vi "Start Sync.vi"(8 "error in (no error)":errorcluster, 10 "current time":timestamp, 11 "gRPC Server in":refnum<class "HVC3.lvclass">) -> (0 "error out":errorcluster, 3 "gRPC Server out":refnum<class "HVC3.lvclass">)   [LabVIEW 2019, in "HVC3.lvlib" / "HVC3.lvclass"]
uses:
  HVC3.lvclass
  RPC Messages/measurementservice_DMMConfigRequest/measurementservice_DMMConfigRequest_Data.ctl
  HVC3.lvclass/HVC3.ctl
  RPC Messages/measurementservice_QueryResponse/measurementservice_QueryResponse_Data.ctl
  RPC Messages/measurementservice_DMMConfigResponse/measurementservice_DMMConfigResponse_Data.ctl
  RPC Messages/measurementservice_ErrorOut/measurementservice_ErrorOut_Data.ctl
  RPC Messages/measurementservice_DMMVoltageData/measurementservice_DMMVoltageData_Data.ctl
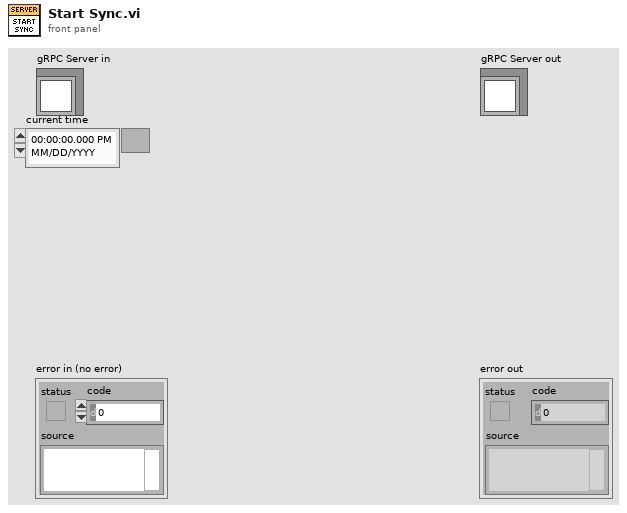
[diagram p1: front panel]
types:
  T1 = typedef "HVC3.lvlib/HVC3.lvclass/measurementservice_DMMConfigRequest_Data.ctl" = cluster{"DMMFunction":i32, "DMMResolution":sgl, "DMMRange":sgl, "DMMSampleCount":i32, "DMMApertureTimeUnit":i32, "DMMApertureTime":sgl, "DMMNumberofAverages":i32, "DMMAutoZero":i32, "DMMADCCalibration":i32, "DMMSettleTime":sgl}
  T2 = cluster{"measurementservice_DMMConfigRequest_Data":T1}
  T3 = typedef "HVC3.lvlib/HVC3.lvclass/measurementservice_QueryResponse_Data.ctl" = cluster{"message":string, "status":i32}
  T4 = typedef "HVC3.lvlib/HVC3.lvclass/measurementservice_ErrorOut_Data.ctl" = cluster{"errCode":i32, "errMessage":string}
  T5 = typedef "HVC3.lvlib/HVC3.lvclass/measurementservice_DMMConfigResponse_Data.ctl" = cluster{"DMMFunction":i32, "DMMResolution":sgl, "DMMRange":sgl, "DMMSampleCount":i32, "DMMApertureTimeUnit":i32, "DMMApertureTime":sgl, "DMMNumberofAverages":i32, "DMMAutoZero":i32, "DMMADCCalibration":i32, "DMMSettleTime":sgl, "error":T4}
  T6 = typedef "HVC3.lvlib/HVC3.lvclass/measurementservice_DMMVoltageData_Data.ctl" = cluster{"voltage":sgl[], "error":T4}
  T7 = typedef "HVC3.lvlib/HVC3.lvclass/Server gRPC UEs.ctl" = cluster{"Invoke gRPC UE":refnum<user-event>, "Query gRPC UE":refnum<user-event>, "Register gRPC UE":refnum<user-event>, "ConfigureDMM gRPC UE":refnum<user-event>, "PerformDMMVoltageMeasurement gRPC UE":refnum<user-event>}
  T8 = typedef "HVC3.lvlib/gprc-lvsupport.lvlib/grpcId.ctl" = u64
  T9 = typedef "HVC3.lvlib/HVC3.lvclass/measurementservice_QueryRequest_Data.ctl" = cluster{"query":string}
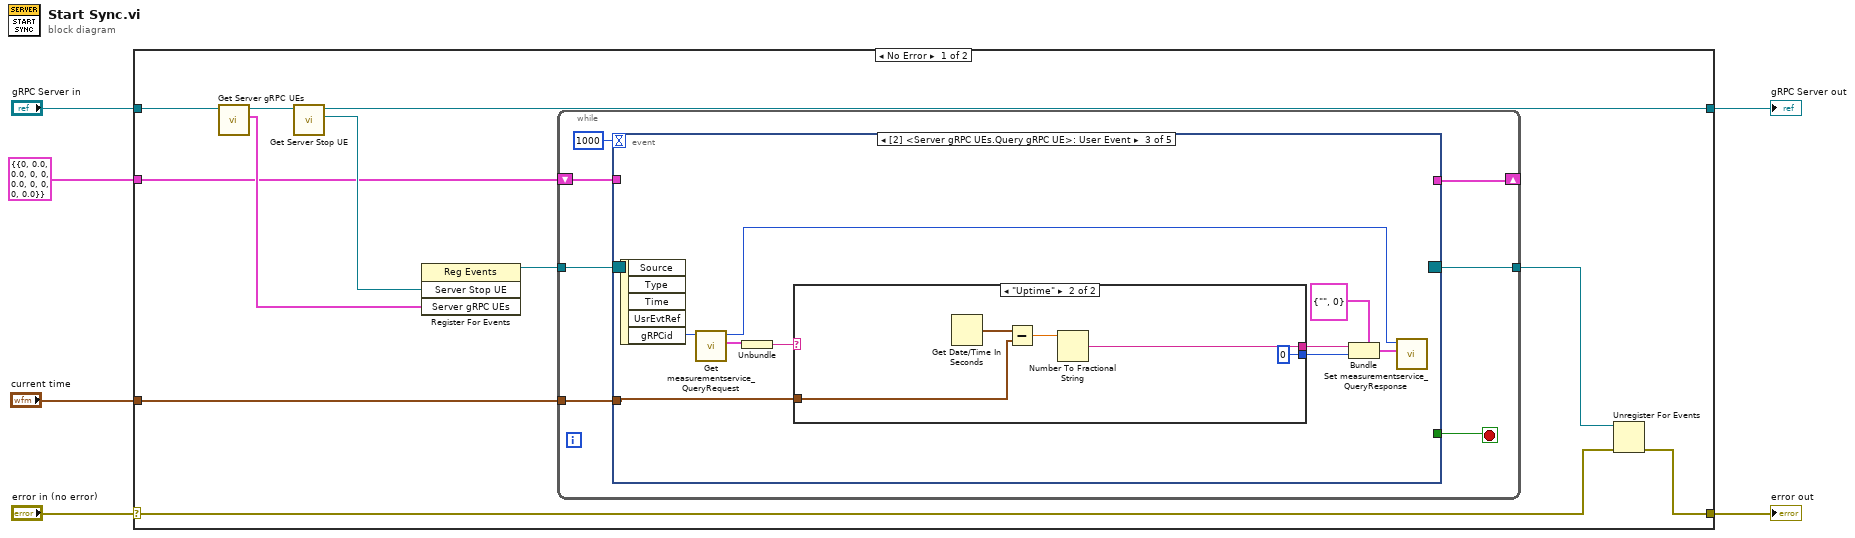
[diagram p0: block diagram]
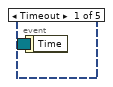
[diagram p2: hidden frame]
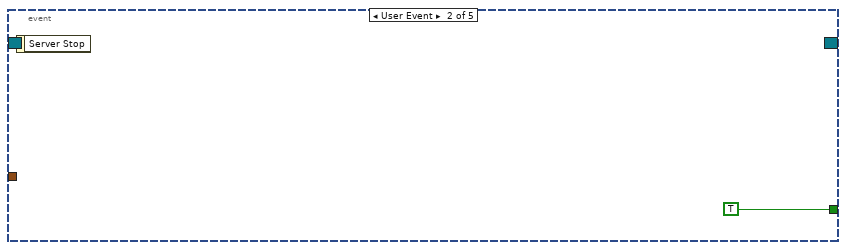
[diagram p3: hidden frame]
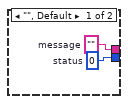
[diagram p4: hidden frame]
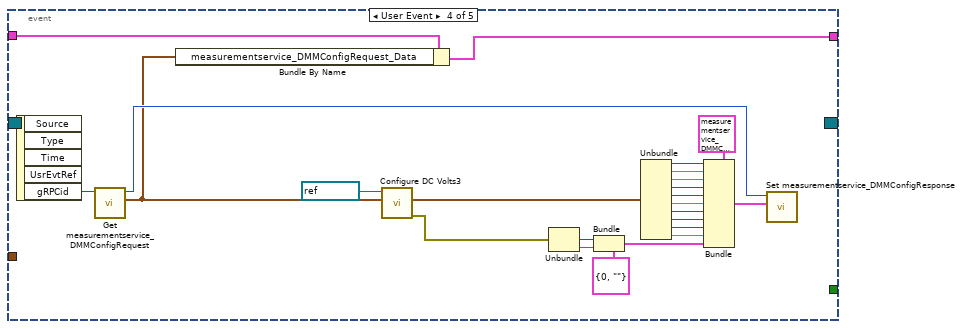
[diagram p5: hidden frame]
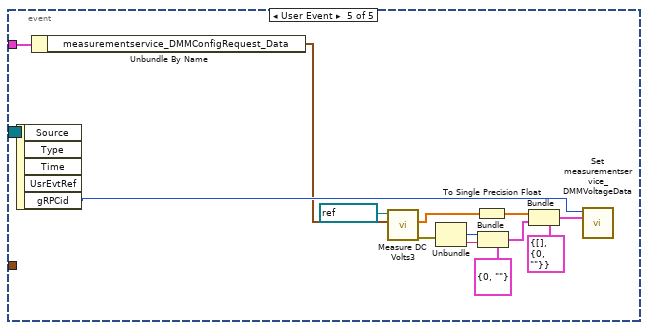
[diagram p6: hidden frame]
diagram:
  n1 = case shown="No Error" "error in (no error)" {
    selector: "error in (no error)" -> [w10 w80]
    tunnel: [w9 w80] -> w5
    tunnel: [w13 w79] -> w3
    tunnel: "gRPC Server in" -> [w17 w79]
    tunnel: "current time" -> [w8 _]
    tunnel: T2 {"measurementservice_DMMConfigRequest_Data"={"DMMFunction"=0, "DMMResolution"=0.0, "DMMRange"=0.0, "DMMSampleCount"=0, "DMMApertureTimeUnit"=0, "DMMApertureTime"=0.0, "DMMNumberofAverages"=0, "DMMAutoZero"=0, "DMMADCCalibration"=0, "DMMSettleTime"=0.0}} -> [w7 _]
    frame No Error {
      n2 = call "Get Server gRPC UEs.vi"("OOP Server in"=w17) -> ("Server gRPC UEs"=w14:T7, "OOP Server out"=w16:refnum<class "HVC3.lvclass">)  [unwired: 9 in]
      n3 = call "Get Server Stop UE.vi"("OOP Server in"=w16) -> ("Server Stop UE"=w15:refnum<user-event>, "OOP Server out"=w13:refnum<class "HVC3.lvclass">)  [unwired: 9 in]
      n4 = register-events(w15, w14) -> (reference out=w12:refnum<event-registration>)  [unwired: 2 in, 1 out]
      n5 = while {
        tunnel: w12 -> [w24]
        tunnel: [w22] -> w11
        tunnel: w8 -> [w20]
        shift-right: [w18] -> _
        shift-left: w7 -> [w19]
        stop <- w23 stop-if-true
        n6 = event "RPC Methods Event Structure" shown="[2] <Server gRPC UEs.Query gRPC UE>: User Event" {
          selector: w24 -> [_ _ _ _ _]
          dyn-events: [_ _ _ _ _] -> w22
          timeout: 1000 -> [_ _ _ _ _]
          tunnel: [_ TRUE _ _ _] -> w23
          tunnel: w20 -> [_ _ w31 _ _]
          tunnel: w19 -> [_ _ _ w52 w78]
          tunnel: [_ _ _ w51 _] -> w18
          event Timeout {
            n7 = event-data() -> ()  [unwired: 1 in, 1 out]
          }
          event User Event {
            n8 = event-data() -> ()  [unwired: 1 in, 1 out]
          }
          event User Event {
            n9 = event-data() -> ("gRPCid"=w30:T8)  [unwired: 1 in, 4 out]
            n10 = call "Get measurementservice_QueryRequest.vi"("gRPCid"=w30) -> ("Message Data"=w29:T9, "gRPCid out"=w27:T8)  [unwired: 8 in, 1 out]
            n11 = Unbundle(w29) -> ("query"=w34:string)
            n12 = case shown="\"Uptime\"" w34 {
              tunnel: [w36 0 ("status")] -> w33
              tunnel: [w35 w39] -> w32
              tunnel: w31 -> [_ w37]
              frame "", Default {
                w35 = ""  # message
                w36 = 0  # status
              }
              frame "Uptime" {
                n13 = Get Date/Time In Seconds() -> (seconds since 1Jan1904=w41:timestamp)
                n14 = Subtract(x=w41, y=w37) -> (x-y=w40:dbl)
                n15 = Number To Fractional String(number=w40) -> (F-format string=w39:string)  [unwired: 3 in]
              }
            }
            n16 = Bundle(cluster=T3 {"message"="", "status"=0} ("measurementservice_QueryResponse_Data"), "message"=w32, "status"=w33) -> (w26:T3)
            n17 = call "Set measurementservice_QueryResponse.vi"("Message Data"=w26, "gRPCid"=w27) -> ()  [unwired: 9 in, 1 out]
          }
          event User Event {
            n18 = event-data() -> ("gRPCid"=w53:T8)  [unwired: 1 in, 4 out]
            n19 = call "Get measurementservice_DMMConfigRequest.vi"("gRPCid"=w53) -> ("Message Data"=w46:T1, "gRPCid out"=w49:T8)  [unwired: 8 in, 1 out]
            n20 = Bundle By Name(cluster=w52, "measurementservice_DMMConfigRequest_Data"=w46) -> (w51:T2)
            n21 = call "Configure DC Volts3.vi"("measurementservice_DMMConfigRequest_Data"=w46, "IVI Refnum in"=refnum<k15> "DMM") -> ("error out"=w44:errorcluster, "measurementservice_DMMConfigRequest_Data Out"=w45:T1)  [unwired: 8 in]
            n22 = Unbundle(w44) -> ("code"=w55:i32, "source"=w54:string)  [unwired: 1 out]
            n23 = Bundle(cluster=T4 {"errCode"=0, "errMessage"=""} ("error"), "errCode"=w55, "errMessage"=w54) -> (w42:T4)
            n24 = Unbundle(w45) -> ("DMMFunction"=w65:i32, "DMMResolution"=w64:sgl, "DMMRange"=w63:sgl, "DMMSampleCount"=w62:i32, "DMMApertureTimeUnit"=w61:i32, "DMMApertureTime"=w60:sgl, "DMMNumberofAverages"=w59:i32, "DMMAutoZero"=w58:i32, "DMMADCCalibration"=w57:i32, "DMMSettleTime"=w56:sgl)
            n25 = Bundle(cluster=T5 {"DMMFunction"=0, "DMMResolution"=0.0, "DMMRange"=0.0, "DMMSampleCount"=0, "DMMApertureTimeUnit"=0, "DMMApertureTime"=0.0, "DMMNumberofAverages"=0, "DMMAutoZero"=0, "DMMADCCalibration"=0, "DMMSettleTime"=0.0, "error"={"errCode"=0, "errMessage"=""}} ("measurementservice_DMMConfigResponse_Data"), "DMMFunction"=w65, "DMMResolution"=w64, "DMMRange"=w63, "DMMSampleCount"=w62, "DMMApertureTimeUnit"=w61, "DMMApertureTime"=w60, "DMMNumberofAverages"=w59, "DMMAutoZero"=w58, "DMMADCCalibration"=w57, "DMMSettleTime"=w56, "error"=w42) -> (w48:T5)
            n26 = call "Set measurementservice_DMMConfigResponse.vi"("Message Data"=w48, "gRPCid"=w49) -> ()  [unwired: 9 in, 1 out]
          }
          event User Event {
            n27 = event-data() -> ("gRPCid"=w77:T8)  [unwired: 1 in, 4 out]
            n28 = Unbundle By Name(w78) -> ("measurementservice_DMMConfigRequest_Data"=w71:T1)
            n29 = call "Measure DC Volts3.vi"("measurementservice_DMMConfigRequest_Data"=w71, "IVI Refnum in"=refnum<k15> "DMM" ("Device Name")) -> ("error out"=w68:errorcluster, "Measurement Array (Volts)"=w70:dbl[])  [unwired: 8 in]
            n30 = Unbundle(w68) -> ("code"=w67:i32, "source"=w66:string)  [unwired: 1 out]
            n31 = To Single Precision Float(number=w70) -> (single precision float=w69:sgl[])
            n32 = Bundle(cluster=T4 {"errCode"=0, "errMessage"=""} ("error"), "errCode"=w67, "errMessage"=w66) -> (w73:T4)
            n33 = Bundle(cluster=T6 {"voltage"=[], "error"={"errCode"=0, "errMessage"=""}} ("Message Data"), "voltage"=w69, "error"=w73) -> (w76:T6)
            n34 = call "Set measurementservice_DMMVoltageData.vi"("Message Data"=w76, "gRPCid"=w77) -> ()  [unwired: 9 in, 1 out]
          }
        }
      }
      n35 = Unregister For Events(event registration refnum=w11, error in=w10) -> (error out=w9:errorcluster)
    }
    frame Error {
    }
  }
  "error out" <- w5
  "gRPC Server out" <- w3
